vi "Top7best.vi"() -> ()   [LabVIEW 2013]
uses:
  <vilib>/Analysis/baseanly.llb/Mean (DBL).vi
  <vilib>/Analysis/NI_AALBase.lvlib
panel:
  in  "?":dbl(slide) scale=2048.0..4096.0
  out "Напряжение на вентиляторе, В":dbl
  out "Ток на вентиляторе, A":dbl
  out "Частота, об/мин":dbl
  out "Частота, об/c":i32
  in  "stop":bool=TRUE
  # "Руководство пользователя"
  # "Измеряемые параметры"
  # "Для регулировки скорости вращения вентилятора измените положение ползунка в блоке \"Регулировка скорости\".\nДля завершения работы программы нажмите на кнопку \"Остановка программы\".\n\nВращение начинается при напряжении ~3В \n(Примерно середина ползунка)"
  # "Регулировка скорости"
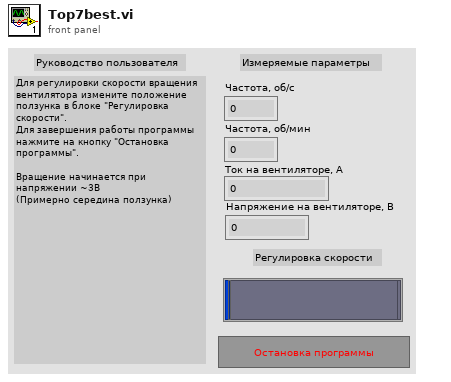
[diagram p1: front panel]
types:
  T1 = enum16{"open", "replace", "create", "open or create", "replace or create", "replace or create with confirmation"}
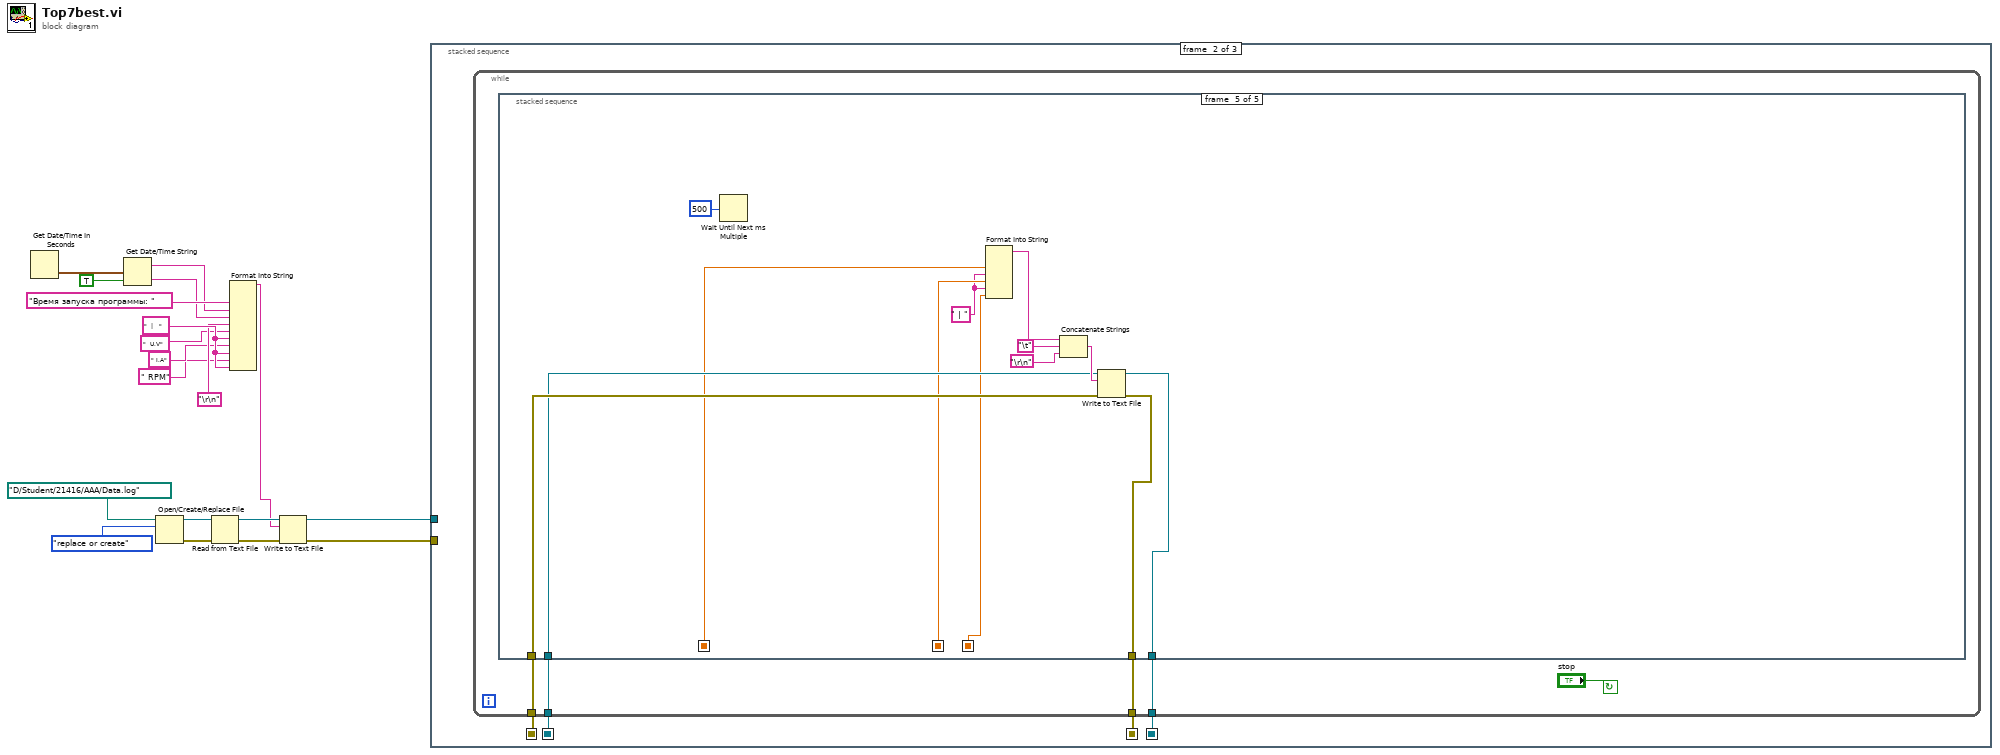
[diagram p0: block diagram]
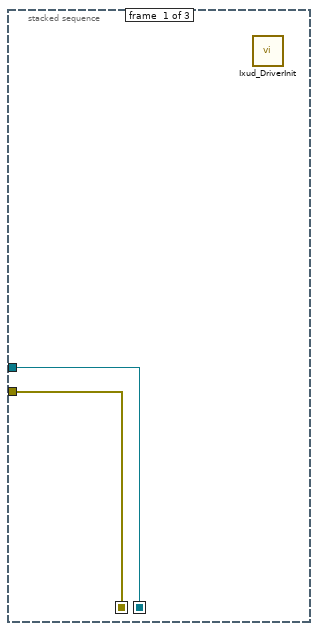
[diagram p2: hidden frame]
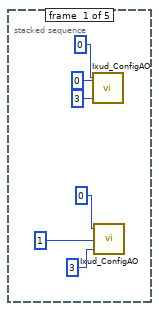
[diagram p3: hidden frame]
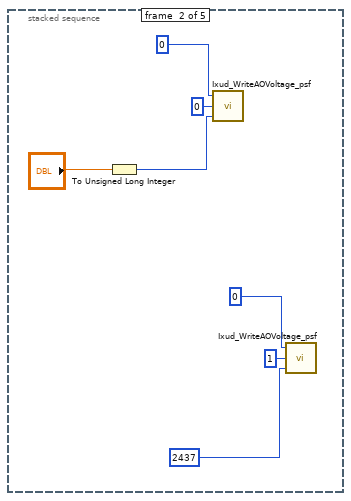
[diagram p4: hidden frame]
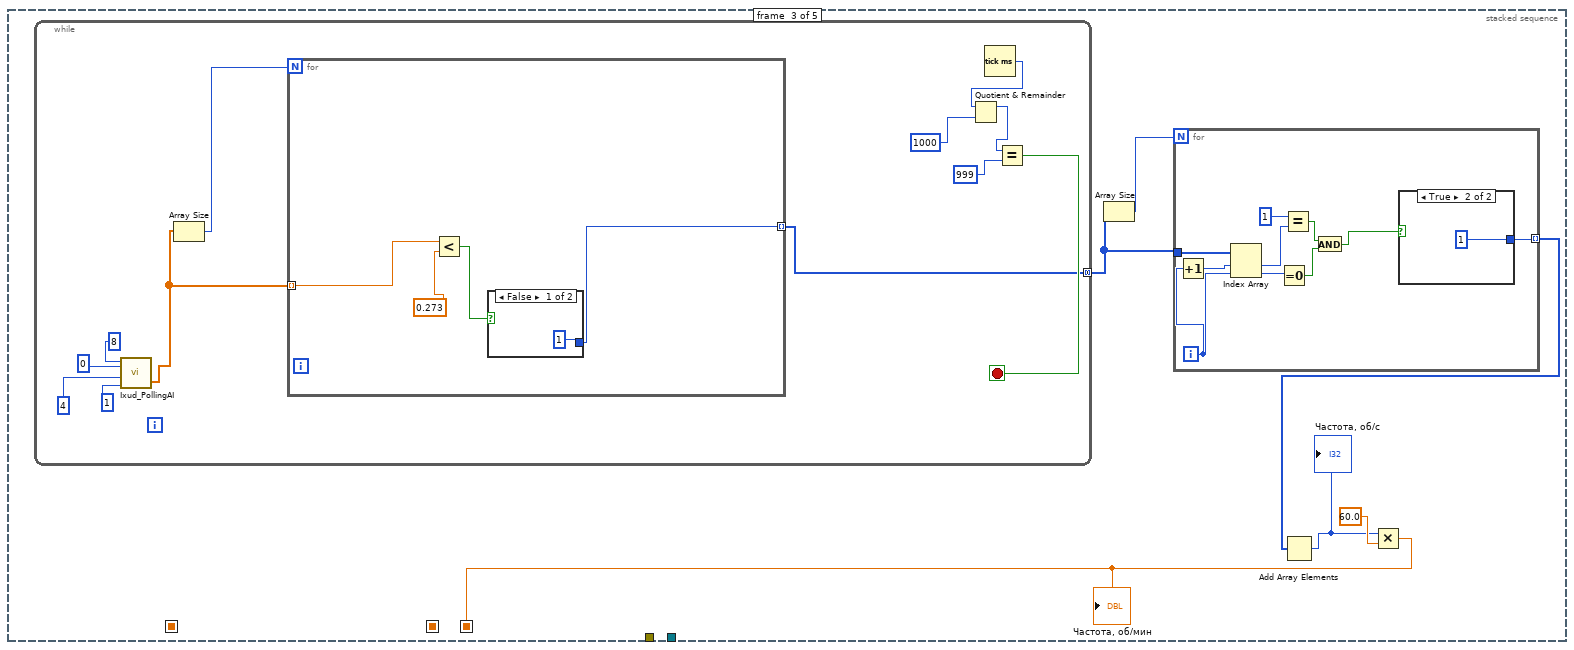
[diagram p5: hidden frame]
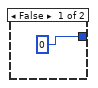
[diagram p6: hidden frame]
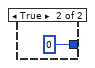
[diagram p7: hidden frame]
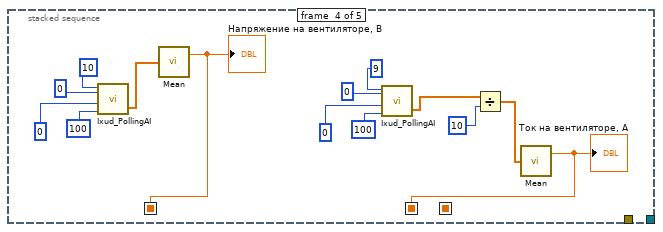
[diagram p8: hidden frame]
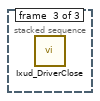
[diagram p9: hidden frame]
diagram:
  w10 = "  |   "
  n1 = Get Date/Time In Seconds() -> (seconds since 1Jan1904=w11:timestamp)
  n2 = Get Date/Time String(seconds (now)=w11, want seconds? (F)=TRUE) -> (date string=w5:string, time string=w6:string)  [unwired: 1 in]
  n3 = Open/Create/Replace File(file path (use dialog)=path "D:/Student/21416/AAA/Data.log", operation (0:open)=T1."replace or create") -> (refnum out=w17:refnum<file>, error out=w16:errorcluster)  [unwired: 4 in, 1 out]
  n4 = Read from Text File(file (use dialog)=w17, error in=w16) -> (refnum out=w19:refnum<file>, error out=w18:errorcluster)  [unwired: 2 in, 2 out]
  n5 = Format Into String("Время запуска программы: " ("input 1"), w5, w6, "\r\n", "  U,V", w10, " I,A" ("input 3"), w10, " RPM" ("input 5"), w10) -> (resulting string=w1:string)  [unwired: 3 in, 1 out]
  n6 = Write to Text File(file (use dialog)=w19, text=w1, error in=w18) -> (refnum out=w12:refnum<file>, error out=w13:errorcluster)  [unwired: 1 in, 1 out]
  n7 = stacked-sequence {
    seq-local: [w21 _ _] -> [_ w25 _]
    seq-local: [w20 _ _] -> [_ w24 _]
    seq-local: [_ w23 _] -> [_ _ _]
    seq-local: [_ w22 _] -> [_ _ _]
    tunnel: w13 -> [w21 _ _]
    tunnel: w12 -> [w20 _ _]
    frame #0 {
      n8 = call "Ixud_DriverInit.vi"() -> ()  [unwired: 2 out]
    }
    frame #1 {
      n9 = while {
        tunnel: w25 -> [w29]
        tunnel: w24 -> [w28]
        tunnel: [w27] -> w23
        tunnel: [w26] -> w22
        stop <- "stop" continue-if-true
        n10 = stacked-sequence {
          seq-local: [_ _ _ w81 _] -> [_ _ _ _ w97]
          seq-local: [_ _ _ w80 _] -> [_ _ _ _ w96]
          seq-local: [_ _ w47 _ _] -> [_ _ _ _ w94]
          tunnel: w29 -> [_ _ _ _ w101]
          tunnel: w28 -> [_ _ _ _ w100]
          tunnel: [_ _ _ _ w99] -> w27
          tunnel: [_ _ _ _ w98] -> w26
          frame #0 {
            n11 = call "Ixud_ConfigAO.vi"("wCfgCode"=u16 3, "wChannel"=u16 0, "wBoardNo"=u16 0) -> ()  [unwired: 1 out]
            n12 = call "Ixud_ConfigAO.vi"("wCfgCode"=u16 3, "wChannel"=u16 1, "wBoardNo"=u16 0) -> ()  [unwired: 1 out]
          }
          frame #1 {
            n13 = To Unsigned Long Integer(number="?") -> (unsigned 32bit integer=w37:u32)
            n14 = call "Ixud_WriteAOVoltage_psf.vi"("Code"=w37, "wChannel"=u16 0, "wBoardNo"=u16 0) -> ()  [unwired: 1 out]
            n15 = call "Ixud_WriteAOVoltage_psf.vi"("Code"=u16 2437 ("AO_CfgCode 2"), "wChannel"=u16 1, "wBoardNo"=u16 0) -> ()  [unwired: 1 out]
          }
          frame #2 {
            n16 = while {
              tunnel: [w62] -> w44 mode=concatenating
              stop <- w65 stop-if-true
              n17 = call "Ixud_PollingAI.vi"("dwDataCount"=u32 1, "wConfig"=u16 4 ("AI_Range"), "wBoardNo"=u16 0, "wChannel"=u16 8 ("AI_Channel")) -> ("fValue"=w64:sgl[])  [unwired: 1 out]
              n18 = Array Size(array=w64) -> (size(s)=w69:i32)
              n19 = for {
                N: w69 -> [_]
                tunnel: [w76] -> w62 mode=indexing
                tunnel: w64 -> [w77] mode=indexing
                n20 = Less?(x=w77, y=0.273) -> (x < y?=w75:bool)
                n21 = case shown="False" w75 {
                  tunnel: [1 0] -> w76
                  frame False {
                  }
                  frame True {
                  }
                }
              }
              n22 = Tick Count (ms)() -> (millisecond timer value=w63:u32)
              n23 = Quotient & Remainder(x=w63, y=1000) -> (x-y*floor(x/y)=w66:u32)  [unwired: 1 out]
              n24 = Equal?(x=w66, y=999) -> (x = y?=w65:bool)
            }
            n25 = Array Size(array=w44) -> (size(s)=w45:i32)
            n26 = for {
              N: w45 -> [_]
              tunnel: w44 -> [w59]
              tunnel: [w52] -> w46 mode=indexing
              i -> [w50]
              n27 = Increment(x=w50) -> (x+1=w51:i32)
              n28 = Index Array(array=w59, index #1=w51, index #2=w50) -> (element #1=w57:i32, element #2=w58:i32)
              n29 = Equal To 0?(x=w58) -> (x = 0?=w54:bool)
              n30 = Equal?(x=1, y=w57) -> (x = y?=w55:bool)
              n31 = And(x=w55, y=w54) -> (x .and. y?=w53:bool)
              n32 = case shown="True" w53 {
                tunnel: [0 1] -> w52
                frame False {
                }
                frame True {
                }
              }
            }
            n33 = Add Array Elements(numeric array=w46) -> (sum=w48:i32)
            "Частота, об/c" <- w48
            n34 = Multiply(x=w48, y=60.0) -> (x*y=w47:dbl)
            "Частота, об/мин" <- w47
          }
          frame #3 {
            n35 = call "Ixud_PollingAI.vi"("dwDataCount"=u32 100, "wConfig"=u16 0 ("AI_Range"), "wBoardNo"=u16 0, "wChannel"=u16 10 ("AI_Channel")) -> ("fValue"=w85:sgl[])  [unwired: 1 out]
            n36 = call-poly <vilib>:"Mean.vi"("X"=w85) -> ("mean"=w81:dbl)  [unwired: 1 out]
            "Напряжение на вентиляторе, В" <- w81
            n37 = call "Ixud_PollingAI.vi"("dwDataCount"=u32 100, "wConfig"=u16 0 ("AI_Range"), "wBoardNo"=u16 0, "wChannel"=u16 9 ("AI_Channel")) -> ("fValue"=w83:sgl[])  [unwired: 1 out]
            n38 = Divide(x=w83, y=10) -> (x/y=w82:sgl[])
            n39 = call-poly <vilib>:"Mean.vi"("X"=w82) -> ("mean"=w80:dbl)  [unwired: 1 out]
            "Ток на вентиляторе, A" <- w80
          }
          frame #4 {
            w95 = " | "
            n40 = Wait Until Next ms Multiple(millisecond multiple=u32 500) -> ()  [unwired: 1 out]
            n41 = Format Into String(w97, w95, w96, w95, w94) -> (resulting string=w103:string)  [unwired: 3 in, 1 out]
            n42 = Concatenate Strings(w103, "\t", "\r\n") -> (w104:string)
            n43 = Write to Text File(file (use dialog)=w100, text=w104, error in=w101) -> (refnum out=w98:refnum<file>, error out=w99:errorcluster)  [unwired: 1 in, 1 out]
          }
        }
      }
    }
    frame #2 {
      n44 = call "Ixud_DriverClose.vi"() -> ()  [unwired: 1 in]
    }
  }
